vi "test I8.vi"(8 "error in (no error)":errorcluster, 11 "TestCase in":refnum<class "Scan From Python String Tests.lvclass">) -> (0 "error out":errorcluster, 3 "TestCase out":refnum<class "Scan From Python String Tests.lvclass">)   [LabVIEW 2020, in "Scan From Python String Tests.lvclass"]
uses:
  Scan From Python String Tests.lvclass
  source/Python String to LabVIEW Data/Python String to LabVIEW Data (I8).vi
  Scan From Python String Tests.lvclass/Scan From Python String Tests.ctl
  <vilib>/addons/_JKI Toolkits/VI Tester/TestCase.llb/TestCase.lvclass
  source/jki_python_data_tools.lvlib
  C:/Program Files/National Instruments/LabVIEW 2020/vi.lib/addons/_JKI Toolkits/VI Tester/TestCase.llb/TestCase.lvclass
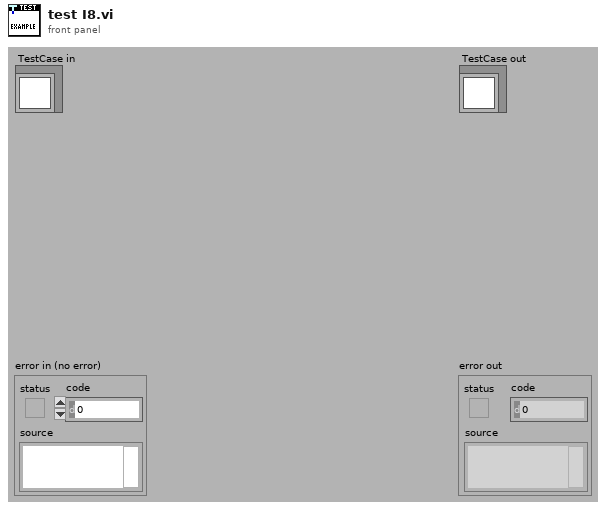
[diagram p1: front panel]
types:
  T1 = cluster{"Input":string, "Expected Result":i8, "Comment":string}
  T2 = cluster{"Input":string, "Expected Result":i8, "Comment":string}[]
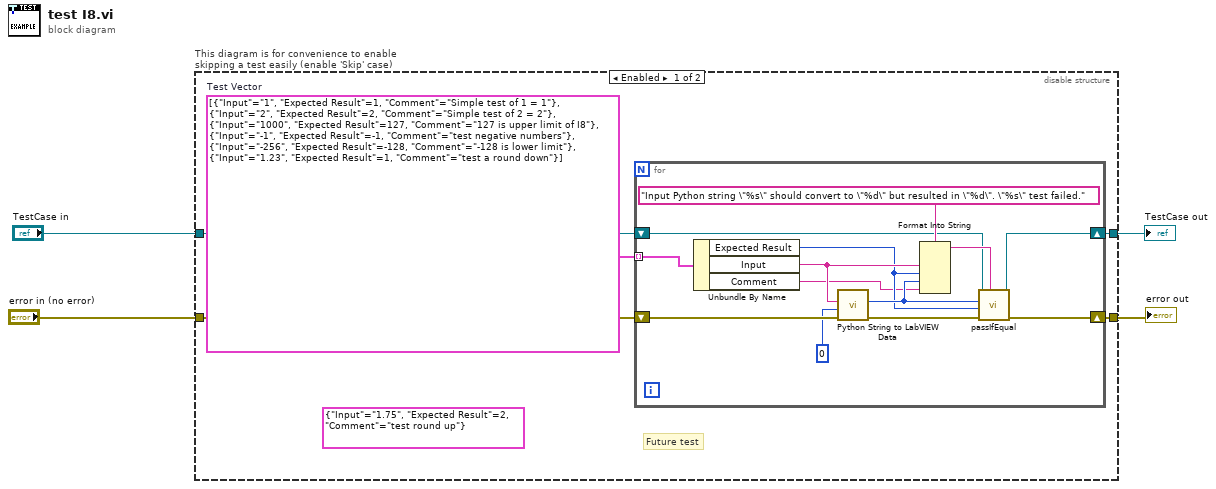
[diagram p0: block diagram]
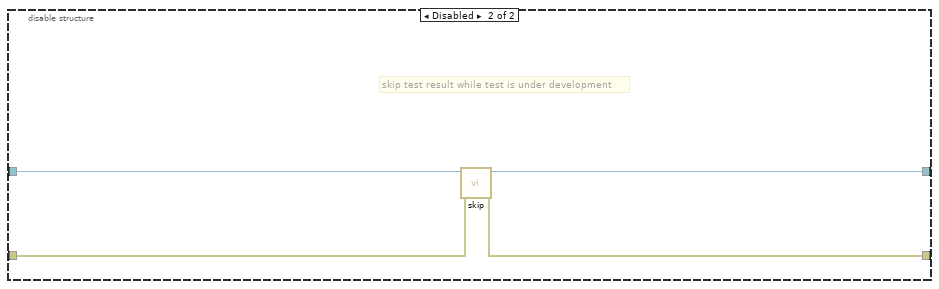
[diagram p2: hidden frame]
diagram:
  n1 = disable-structure "This diagram is for convenience to enable skipping a test easily (enable 'Skip' case)" shown="Enabled" {
    disable-tunnel: "TestCase in" -> [w6 w26]
    disable-tunnel: [w5 w24] -> w1
    disable-tunnel: [w7 w25] -> w3
    disable-tunnel: "error in (no error)" -> [w9 w23]
    frame Enabled {
      (unwired) T1 {"Input"="1.75", "Expected Result"=2, "Comment"="test round up"}
      w8 = T2 [{"Input"="1", "Expected Result"=1, "Comment"="Simple test of 1 = 1"}, {"Input"="2", "Expected Result"=2, "Comment"="Simple test of 2 = 2"}, {"Input"="1000", "Expected Result"=127, "Comment"="127 is upper limit of I8"}, {"Input"="-1", "Expected Result"=-1, "Comment"="test negative numbers"}, {"Input"="-256", "Expected Result"=-128, "Comment"="-128 is lower limit"}, {"Input"="1.23", "Expected Result"=1, "Comment"="test a round down"}]  # Test Vector
      # "Future test"
      n2 = for {
        tunnel: w8 -> [w21] mode=indexing
        shift-right: [w19] -> w7
        shift-left: w9 -> [w22]
        shift-right: [w13] -> w5
        shift-left: w6 -> [w14]
        n3 = Unbundle By Name(w21) -> ("Expected Result"=w12:i8, "Input"=w17:string, "Comment"=w11:string)
        n4 = call-poly "Python String to LabVIEW Data.vi"("error in (no error)"=w22, "type (I8)"=i8 0 ("Default Value"), "Python String"=w17) -> ("error out"=w20:errorcluster, "LabVIEW Data"=w16:i8)  [unwired: 7 in]
        n5 = Format Into String(format string="Input Python string \"%s\" should convert to \"%d\" but resulted in \"%d\". \"%s\" test failed.", w17, w12, w16, w11) -> (resulting string=w18:string)  [unwired: 2 in, 1 out]
        n6 = call-dynamic "passIfEqual.vi"("custom report message (\"\")"=w18, "error in (no error)"=w20, "y"=w12, "x"=w16, "TestCase in"=w14) -> ("error out"=w19:errorcluster, "TestCase out"=w13:refnum<class "Scan From Python String Tests.lvclass">)  [unwired: 5 in]
      }
    }
    frame Disabled {
      # "skip test result while test is under development"
      n7 = call <vilib>:"skip.vi"("error in (no error)"=w23, "TestCase in"=w26) -> ("error out"=w25:errorcluster, "TestCase out"=w24:refnum<class "Scan From Python String Tests.lvclass">)  [unwired: 8 in]
    }
  }
  "error out" <- w3
  "TestCase out" <- w1
